vi "Clear Hardware.vi"(2 "error in (no error)":errorcluster, 3 "Arduino DDS in":refnum<class "Arduino DDS.lvclass">) -> (0 "error out":errorcluster, 1 "Arduino DDS out":refnum<class "Arduino DDS.lvclass">)   [LabVIEW 2013, in "Arduino DDS.lvclass"]
doc: "This VI resets any necessary hardware so that the device will be ready for the next run."
uses:
  Arduino DDS.lvclass
  Device/Device.lvclass
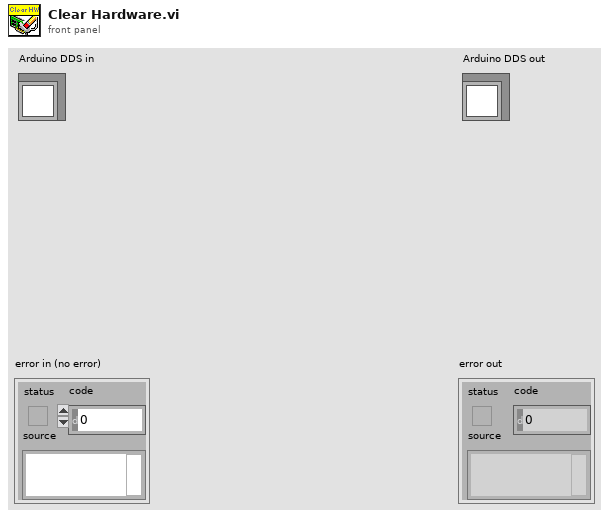
[diagram p1: front panel]
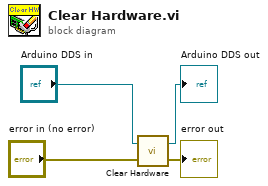
[diagram p0: block diagram]
diagram:
  n1 = call-parent "Clear Hardware.vi"("error in (no error)"="error in (no error)", "Device in"="Arduino DDS in") -> ("error out"=→"error out":errorcluster, "Device out"=→"Arduino DDS out":refnum<class "Arduino DDS.lvclass">)
